vi "多参数启动参数对话框.vi"() -> (2 "确认":bool, 3 "测量时间":dbl)   [LabVIEW 2016, in "斯坦道多参数.lvlib"]
panel:
  in  "time":dbl=3.0
  in  "取消":bool
  in  "确定":bool
  # "请输入测量时间"
  # "min"
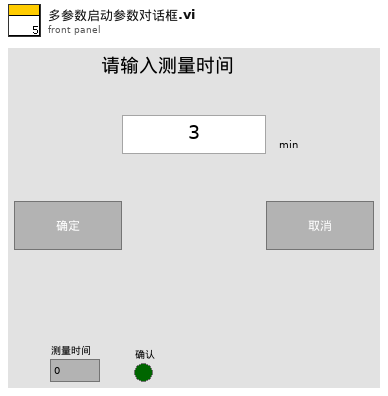
[diagram p1: front panel]
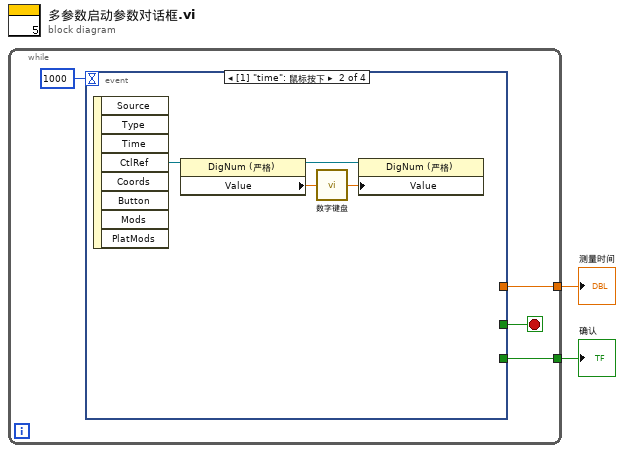
[diagram p0: block diagram]
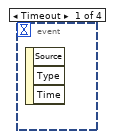
[diagram p2: hidden frame]
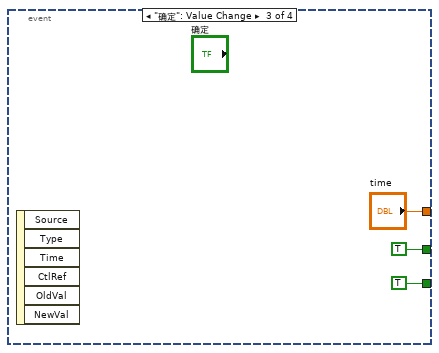
[diagram p3: hidden frame]
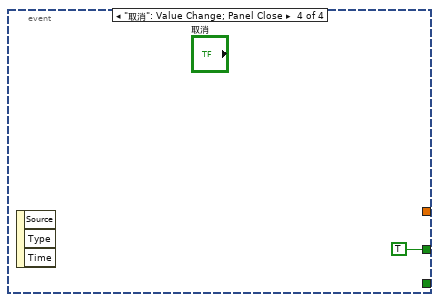
[diagram p4: hidden frame]
diagram:
  n1 = while {
    tunnel: [w4] -> w2
    tunnel: [w3] -> w1
    stop <- w6 stop-if-true
    n2 = event shown="[1] \"time\": 鼠标按下" {
      selector: _ -> [_ _ _ _]
      dyn-events: _ -> [_ _ _ _]
      timeout: 1000 -> [_ _ _ _]
      tunnel: [_ _ TRUE TRUE] -> w6
      tunnel: [_ _ TRUE _] -> w4
      tunnel: [_ _ "time" _] -> w3
      event Timeout {
        n3 = event-data() -> ()  [unwired: 1 in, 3 out]
      }
      event "time": Mouse Down {
        n4 = event-data() -> ("CtlRef"=w10:refnum<vi>)  [unwired: 1 in, 7 out]
        n5 = property class="DigNum (严格)"(reference=w10) -> (reference out=w8:refnum<vi>, "Value"=w9:dbl)  [unwired: 1 in, 1 out]
        n6 = call "数字键盘.vi"("OldNumber"=w9) -> ("NewNumber"=w7:dbl)
        n7 = property class="DigNum (严格)"(reference=w8, "Value"=w7) -> ()  [unwired: 1 in, 2 out]
      }
      event "确定": Value Change {
        n8 = event-data() -> ()  [unwired: 1 in, 6 out]
      }
      event "取消": Value Change; Panel Close {
        n9 = event-data() -> ()  [unwired: 1 in, 3 out]
      }
    }
  }
  "确认" <- w2
  "测量时间" <- w1
